vi "Heartbeat Blinker.vi"(7 "Blink Period [ms]":u32=300, 8 "Error In":errorcluster, 10 "DO Channel":u8=13, 11 "LINX Resource":T1) -> (0 "Error Out":errorcluster, 2 "LED":bool, 3 "LINX Resource Out":T1)   [LabVIEW 2019, in "LINXx.lvlib"]
doc: "Keepalive indicator periodically toggles a digital pin (default onboard LED)"
uses:
  LINXx.lvlib
  <vilib>/MakerHub/LINX/Private/Type Defs/LINX Ref.ctl
  <vilib>/MakerHub/LINX/Private/Type Defs/Platform.ctl
  <vilib>/MakerHub/LINX/Private/Type Defs/Interface.ctl
  <vilib>/MakerHub/LINX/Private/Device/Type Defs/LINX Device Config.ctl
  <vilib>/MakerHub/LINX/Private/Device/Type Defs/TCP Config.ctl
  <vilib>/MakerHub/LINX/Private/Device/Type Defs/Channels.ctl
  <vilib>/MakerHub/LINX/Public/Peripherals/Digital/Digital Write 1 Chan.vi
  <vilib>/MakerHub/LINX/Public/Peripherals/Digital/Digital Write N Chans.vi
  <vilib>/MakerHub/LINX/Private/Local IO/LinxDigitalWrite.vi
  <vilib>/MakerHub/LINX/Public/Utilities/Check Channel.vi
  <vilib>/MakerHub/LINX/Private/Utilties/Generate Error.vi
  <vilib>/MakerHub/LINX/LMH-LINX.lvlib
  <vilib>/MakerHub/LINX/Private/Device/Device.lvlib
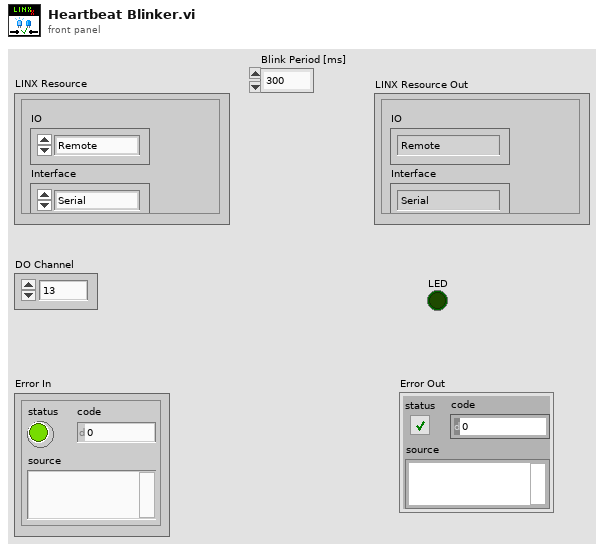
[diagram p1: front panel]
types:
  T1 = typedef "LMH-LINX.lvlib/LINX Ref.ctl" = cluster{"IO":T2, "Interface":T3, "LINX Device Config":T4}
  T2 = typedef "LMH-LINX.lvlib/Platform.ctl" = enum16{"Remote", "Local"}
  T3 = typedef "LMH-LINX.lvlib/Interface.ctl" = enum16{"Serial", "TCP"}
  T4 = typedef "LMH-LINX.lvlib/Device.lvlib/LINX Device Config.ctl" = cluster{"Interface":T3, "COM Port":refnum<visa-resource-name>, "TCP Configuration":T5, "Device Family":u8, "Device ID":u8, "Device Name":string, "TCP Ref":refnum<k5>, "Channels":T6}
  T5 = typedef "LMH-LINX.lvlib/Device.lvlib/TCP Config.ctl" = cluster{"IP Address":string, "Port":u16}
  T6 = typedef "LMH-LINX.lvlib/Channels.ctl" = cluster{"DI":u8[], "DO":u8[], "AI":u8[], "AO":u8[], "PWM":u8[], "QE":u8[], "UART":u8[], "I2C 2":u8[], "SPI":u8[], "CAN":u8[], "Servo":u8[], "AI Ref (V)":dbl, "AI Resolution (Bits)":u8, "AO Ref (V)":dbl, "AO Resolution (Bits)":u8}
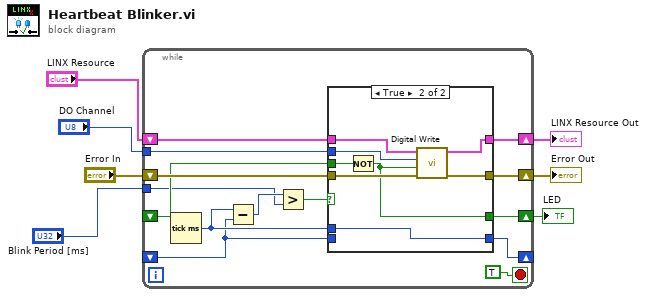
[diagram p0: block diagram]
diagram:
  n1 = while {
    tunnel: "DO Channel" -> [w21]
    shift-right: [w17] -> w2
    shift-left: "Error In" -> [w19]
    shift-right: [w18] -> w3
    shift-left: "LINX Resource" -> [w20]
    shift-right: [w15] -> _
    shift-left: _ -> [w11]
    shift-right: [w14] -> w1
    shift-left: _ -> [w13]
    tunnel: "Blink Period [ms]" -> [w9]
    stop <- TRUE stop-if-true
    n2 = Tick Count (ms)() -> (millisecond timer value=w12:u32)
    n3 = Subtract(x=w12, y=w11) -> (x-y=w10:u32)
    n4 = Greater?(x=w10, y=w9) -> (0:w8:bool)
    n5 = case shown="True" w8 {
      tunnel: w21 -> [_ w33]
      tunnel: w20 -> [w25 w32]
      tunnel: w19 -> [w24 w31]
      tunnel: [w25 w30] -> w18
      tunnel: [w24 w29] -> w17
      tunnel: [w23 w28] -> w15
      tunnel: w12 -> [_ w28]
      tunnel: w11 -> [w23 _]
      tunnel: [w22 w27] -> w14
      tunnel: w13 -> [w22 w26]
      frame False {
      }
      frame True {
        n6 = Not(x=w26) -> (.not. x?=w27:bool)
        n7 = call-poly <vilib>:"Digital Write.vi"("Error In"=w31, "Output Value"=w27, "DO Channel"=w33, "LINX Resource"=w32) -> ("Error Out"=w29:errorcluster, "LINX Resource"=w30:T1)  [unwired: 6 in]
      }
    }
  }
  "LINX Resource Out" <- w3
  "Error Out" <- w2
  "LED" <- w1
